vi "Module Init.vi"(8 "error in (no error)":errorcluster, 11 "DAQmxDI in":refnum<class " DAQmxDI Port.lvclass">) -> (0 "error out":errorcluster, 3 "DAQmxDI out":refnum<class " DAQmxDI Port.lvclass">)   [LabVIEW 2020, in " DAQmxDI Port.lvclass"]
uses:
   DAQmxDI Port.lvclass
   DAQmxDI Port.lvclass/ DAQmxDI Port.ctl
  Volatus/Module/Module.lvclass
  VolatusData/Data Processor Module/Data Processor Module.lvclass
  VolatusDAQ.lvlib
  C:/dev/lv20CE/relink/lv-volatus/Volatus/Module/Module.lvclass
  C:/dev/lv20CE/relink/lv-volatus/VolatusDAQ/DAQmxDI Port/ DAQmxDI Port.lvclass
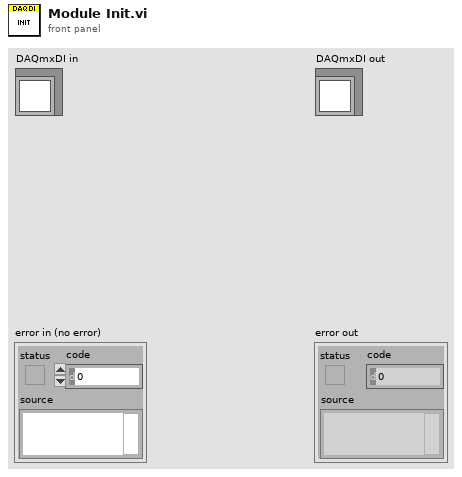
[diagram p1: front panel]
types:
  T1 = typedef "VolatusDAQConfig.lvlib/Sampling Config.ctl" = cluster{"Rate":dbl, "Chunk Size":i32}
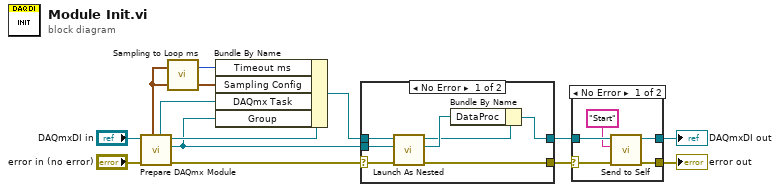
[diagram p0: block diagram]
diagram:
  n1 = call "Prepare DAQmx Module.vi"("error in (no error)"="error in (no error)", "Module in"="DAQmxDI in") -> ("error out"=w9:errorcluster, "Group"=w7:refnum<class "Group DBL.lvclass">, "Module out"=w11:refnum<class " DAQmxDI Port.lvclass">, "DAQmx Task"=w8:refnum<k21>, "Sampling Config"=w2:T1)  [unwired: 4 in, 1 out]
  n2 = call "Sampling to Loop ms.vi"("Sampling Config"=w2) -> ("Loop Timeout ms"=w1:i32)  [unwired: 6 in]
  n3 = Bundle By Name(cluster=w11, "Timeout ms"=w1, "Sampling Config"=w2, "DAQmx Task"=w8, "Group"=w7) -> (w10:refnum<class " DAQmxDI Port.lvclass">)
  n4 = case shown="No Error" w9 {
    selector: w9 -> [w19 w21]
    tunnel: w10 -> [w20 w22]
    tunnel: [w15 w21] -> w13
    tunnel: [w16 w22] -> w12
    tunnel: w7 -> [w14 _]
    frame No Error {
      n5 = call "Launch As Nested.vi"("error in (no error)"=w19, "Group"=w14, "Parent in"=w20) -> ("error out"=w15:errorcluster, "MessageQ"=w18:refnum<class "MessageQ.lvclass">, "Parent in"=w17:refnum<class " DAQmxDI Port.lvclass">)  [unwired: 6 in]
      n6 = Bundle By Name(cluster=w17, "DataProc"=w18) -> (w16:refnum<class " DAQmxDI Port.lvclass">)
    }
    frame Error {
    }
  }
  n7 = case shown="No Error" w13 {
    selector: w13 -> [w27 w29]
    tunnel: [w26 w29] -> w3
    tunnel: w12 -> [w25 w28]
    tunnel: [w24 w28] -> w4
    frame No Error {
      n8 = call "Send to Self.vi"("error in (no error)"=w27, "Message ID"="Start", "Module in"=w25) -> ("error out"=w26:errorcluster, "Module in"=w24:refnum<class " DAQmxDI Port.lvclass">)  [unwired: 7 in]
    }
    frame Error {
    }
  }
  "error out" <- w3
  "DAQmxDI out" <- w4
